vi "Configure Hardware.vi"(8 "error in (no error)":errorcluster, 11 "Hardware Resources in":T1) -> (0 "error out":errorcluster, 3 "Hardware Resources out":T1)   [LabVIEW 2013, in "Acquisition.lvlib"]
doc: "Configure the hardware."
uses:
  Acquisition.lvlib
  Hardware Configuration.ctl
  C:/Program Files (x86)/National Instruments/LabVIEW 2013/vi.lib/ULx/ULx_LV.dll
  <vilib>/ULx/Create Channel.llb/ULx Create Channel (AI-Voltage-Basic).vi
  <vilib>/ULx/Timing.llb/ULx Timing (Sample Clock).vi
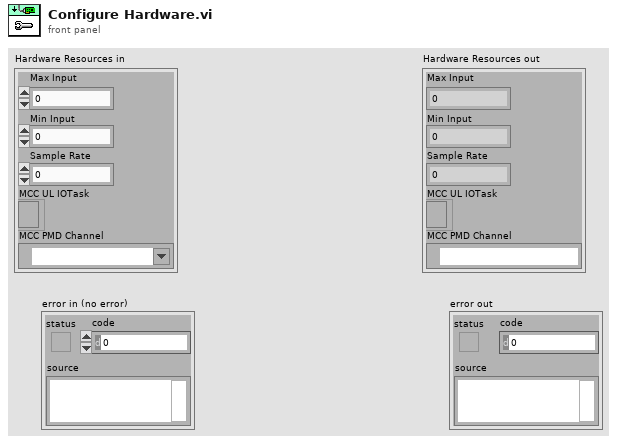
[diagram p1: front panel]
types:
  T1 = typedef "Acquisition.lvlib/Hardware Configuration.ctl" = cluster{"Max Input":dbl, "Min Input":dbl, "Sample Rate":dbl, "MCC UL IOTask":refnum<k24>, "MCC PMD Channel":refnum<k21>}
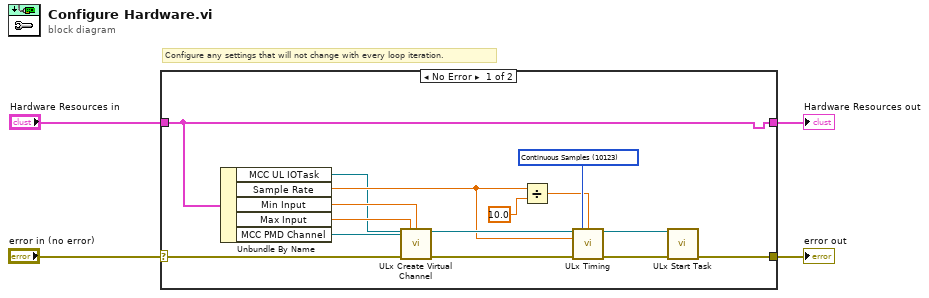
[diagram p0: block diagram]
diagram:
  # "Configure any settings that will not change with every loop iteration."
  n1 = case shown="No Error" "error in (no error)" {
    selector: "error in (no error)" -> [w15 w20]
    tunnel: [w8 w20] -> w3
    tunnel: "Hardware Resources in" -> [w5 w21]
    tunnel: [w5 w21] -> w1
    frame No Error {
      w14 = 10123 items=["Finite Samples"=10178, "Continuous Samples"=10123, "Hardware Timed Single Point"=12522] ("sample mode")
      n2 = Unbundle By Name(w5) -> ("MCC UL IOTask"=w7:refnum<k24>, "Sample Rate"=w13:dbl, "Min Input"=w18:dbl, "Max Input"=w19:dbl, "MCC PMD Channel"=w6:refnum<k21>)
      n3 = call-poly <vilib>:"ULx Create Virtual Channel.vi"("task in"=w7, "maximum value"=w19, "minimum value"=w18, "physical channels"=w6, "error in"=w15) -> ("task out"=w17:refnum<k24>, "error out"=w16:errorcluster)  [unwired: 9 in]
      n4 = Divide(x=w13, y=10.0) -> (x/y=w11:dbl)
      n5 = call-poly <vilib>:"ULx Timing.vi"("task in"=w17, "sample mode"=w14, "samples per channel"=w11, "rate"=w13, "error in"=w16) -> ("task out"=w9:refnum<k24>, "error out"=w10:errorcluster)  [unwired: 9 in]
      n6 = call <vilib>:"ULx Start Task.vi"("task in"=w9, "error in"=w10) -> ("error out"=w8:errorcluster)  [unwired: 12 in, 1 out]
    }
    frame Error {
    }
  }
  "Hardware Resources out" <- w1
  "error out" <- w3
